vi "Test Bench v19 - prep.vi"(6 "Signal Output\nControl":enum32{"White Noise", "Harmonic"}(tab), 8 "Enable Display":bool=TRUE, 9 "Accel. 2":bool, 10 "Output":bool=TRUE) -> (2 "Accel. 1 Raw":dbl[](graph), 3 "Output Signal":dynamicdata(graph))   [LabVIEW 2022 SP3]
uses:
  <vilib>/Utility/error.llb/DialogType.ctl
  <vilib>/DAQmx/create/channels.llb/DAQmx Create Channel (AI-Acceleration-Accelerometer).vi
  <vilib>/DAQmx/create/channels.llb/DAQmx Create Channel (AO-Voltage-Basic).vi
  <vilib>/DAQmx/configure/timing.llb/DAQmx Timing (Sample Clock).vi
  <vilib>/DAQmx/miscellaneous.llb/DAQmx Fill In Error Info.vi
  WhiteNoise.ctl
  <vilib>/DAQmx/write.llb/DAQmx Write (Analog 2D DBL NChan NSamp).vi
  <vilib>/DAQmx/read.llb/DAQmx Read (Analog 1D DBL 1Chan NSamp).vi
  <vilib>/measure/NI_MABase.lvlib
panel:
  out "Input Data":dbl[](array[numeric])
  out "Output Data":dbl[](array[numeric])
  in  "White Noise\nParameters":T2={"Seed"=0.0, "Standard Deviation"=0.2, "Reset"=FALSE, "Iterator"=1.0, "Seed"=-1, "Lower Cut-Off"=5.0, "Upper Cut-Off"=350.0} {"Upper Cut-Off" min=5.0 max=350.0 step=10.0; "Lower Cut-Off" min=5.0 max=350.0 step=10.0; "Standard Deviation" min=0.001 max=3.0 step=0.05 format="%0.2p"}
  in  "Hamonic\nParameters":T3={"Waveform Type"=0, "Frequency"=10.0, "Amplitude"=0.25} {"Frequency" min=5.0 max=350.0 step=10.0 format="%0.2p"; "Waveform Type" items=["Sine Wave", "Triangle Wave", "Square Wave", "Sawtooth Wave"]; "Amplitude" min=0.001 max=0.3 step=0.05 format="%0.2p"}
  # "Filter"
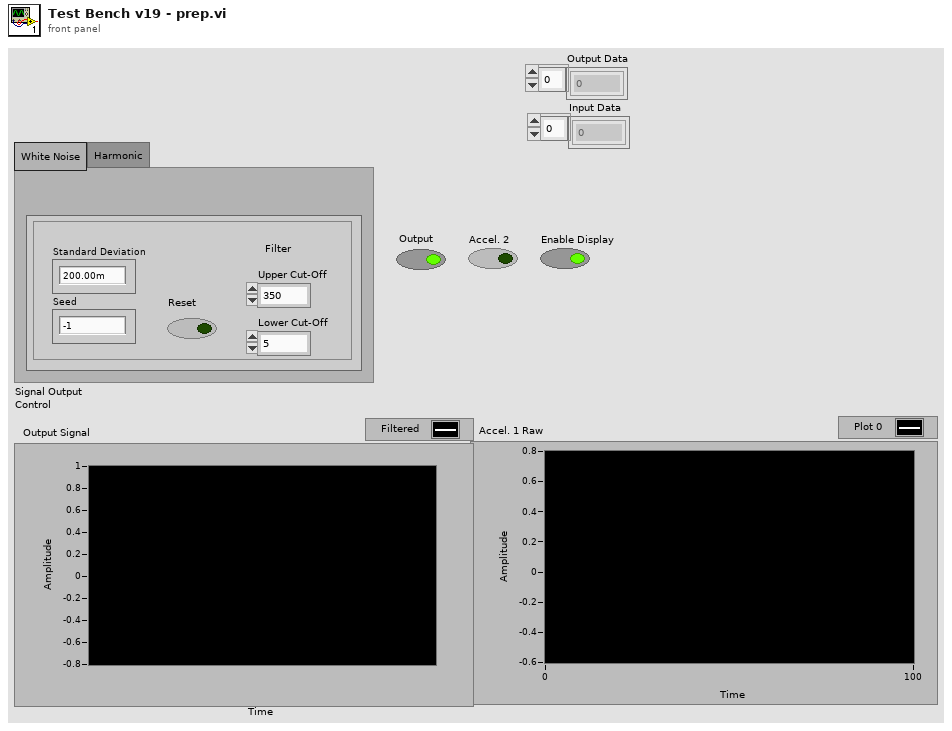
[diagram p1: front panel]
types:
  T1 = typedef "WhiteNoise.ctl" = dbl
  T2 = cluster{"Seed":T1, "Standard Deviation":dbl, "Reset":bool, "Iterator":dbl, "Seed":i8, "Lower Cut-Off":dbl, "Upper Cut-Off":dbl}
  T3 = cluster{"Waveform Type":u16, "Frequency":dbl, "Amplitude":dbl}
  T4 = typedef "DialogType.ctl" = u16
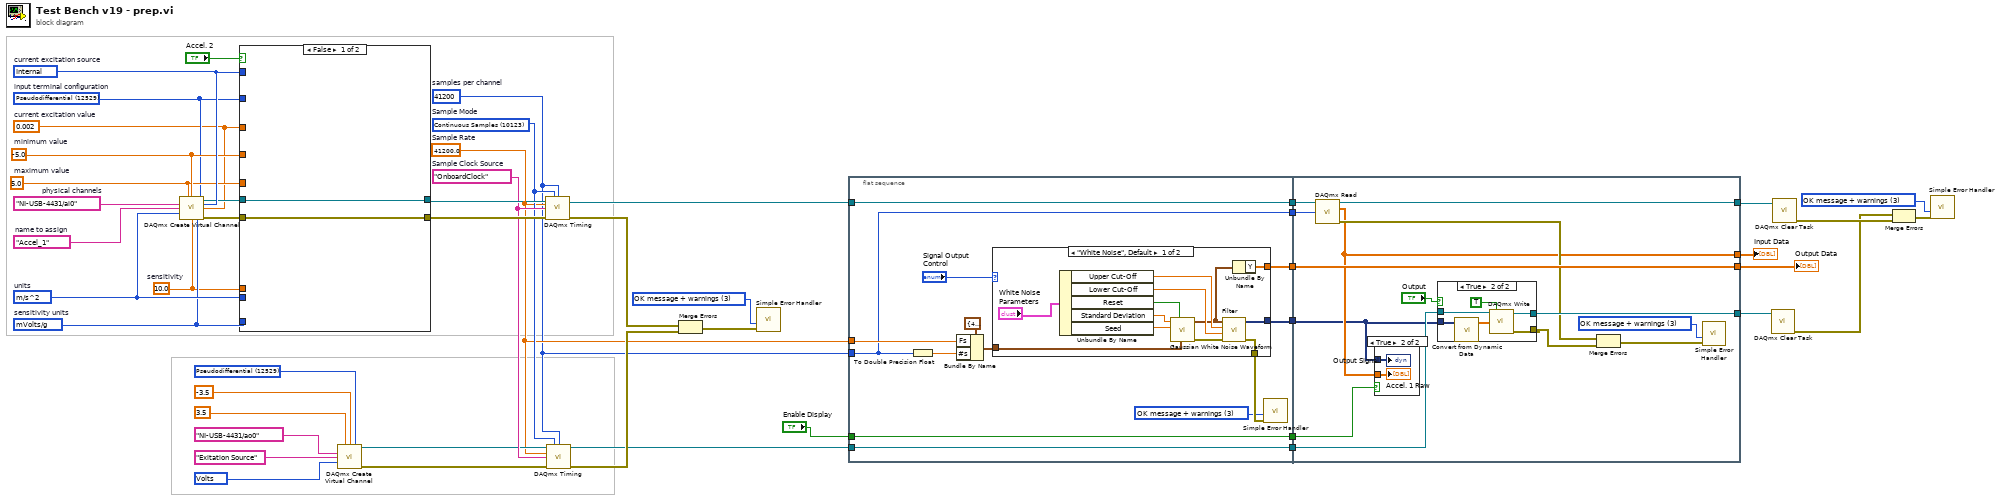
[diagram p0: block diagram]
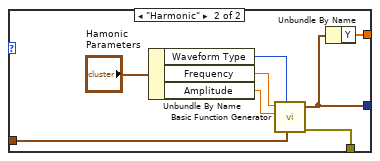
[diagram p2: hidden frame]
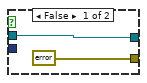
[diagram p4: hidden frame]
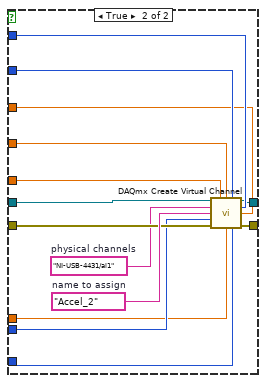
[diagram p5: hidden frame]
diagram:
  w9 = T4 3 items=["no dialog", "OK message", "continue or stop message", "OK message + warnings", "continue/stop + warnings"] ("type of dialog (OK msg:1)")
  w19 = T4 3 items=["no dialog", "OK message", "continue or stop message", "OK message + warnings", "continue/stop + warnings"] ("type of dialog (OK msg:1)")
  w15 = 41200  # samples per channel
  w35 = 12529 items=["Default"=-1, "RSE"=10083, "Differential"=10106, "Pseudodifferential"=12529] ("output terminal configuration")
  w33 = 10348 items=["Volts"=10348, "From Custom Scale"=10065] ("units")
  w39 = 12509 items=["mVolts/g"=12509, "Volts/g"=12510]  # sensitivity units
  w30 = 10.0  # sensitivity
  w38 = 0.002  # current excitation value
  w46 = 10200 items=["Internal"=10200, "External"=10167, "None"=10230]  # current excitation source
  w40 = tag "NI-USB-4431/ai0"  # physical channels
  w27 = tag "OnboardClock"  # Sample Clock Source
  w16 = 41200.0  # Sample Rate
  w26 = 10123 items=["Finite Samples"=10178, "Continuous Samples"=10123, "Hardware Timed Single Point"=12522]  # Sample Mode
  w42 = 12529 items=["default"=-1, "RSE"=10083, "NRSE"=10078, "Differential"=10106, "Pseudodifferential"=12529]  # input terminal configuration
  w45 = -5.0  # minimum value
  w44 = 5.0  # maximum value
  w48 = "Accel_1"  # name to assign
  w43 = 12470 items=["g"=10186, "m/s^2"=12470, "in/s^2"=12471, "From Custom Scale"=10065]  # units
  n1 = call-poly <vilib>:"DAQmx Create Virtual Channel.vi"("maximum value"=w44, "minimum value"=w45, "input terminal configuration"=w42, "physical channels"=w40, "current excitation source"=w46, "name to assign"=w48, "current excitation value"=w38, "units"=w43, "sensitivity"=w30, "sensitivity units"=w39) -> ("task out"=w41:refnum<k21>, "error out"=w47:errorcluster)  [unwired: 4 in]
  n2 = case shown="False" "Accel. 2" {
    tunnel: w47 -> [w50 w63]
    tunnel: w46 -> [_ w62]
    tunnel: w45 -> [_ w61]
    tunnel: w44 -> [_ w60]
    tunnel: w43 -> [_ w59]
    tunnel: w42 -> [_ w58]
    tunnel: w41 -> [w49 w57]
    tunnel: w39 -> [_ w55]
    tunnel: w38 -> [_ w54]
    tunnel: w30 -> [_ w53]
    tunnel: [w50 w52] -> w29
    tunnel: [w49 w51] -> w28
    frame False {
    }
    frame True {
      w56 = tag "NI-USB-4431/ai1"  # physical channels
      w64 = "Accel_2"  # name to assign
      n3 = call-poly <vilib>:"DAQmx Create Virtual Channel.vi"("task in"=w57, "maximum value"=w60, "minimum value"=w61, "input terminal configuration"=w58, "physical channels"=w56, "current excitation source"=w62, "name to assign"=w64, "current excitation value"=w54, "units"=w59, "error in"=w63, "sensitivity"=w53, "sensitivity units"=w55) -> ("task out"=w51:refnum<k21>, "error out"=w52:errorcluster)  [unwired: 2 in]
    }
  }
  n4 = call-poly <vilib>:"DAQmx Create Virtual Channel.vi"("maximum value"=3.5, "minimum value"=-3.5, "output terminal configuration"=w35, "physical channels"=tag "NI-USB-4431/ao0", "name to assign"="Exitation Source", "units"=w33) -> ("task out"=w24:refnum<k21>, "error out"=w25:errorcluster)  [unwired: 8 in]
  n5 = call-poly <vilib>:"DAQmx Timing.vi"("task/channels in"=w28, "sample mode"=w26, "samples per channel"=w15, "rate"=w16, "source"=w27, "error in"=w29) -> ("task out"=w18:refnum<k21>, "error out"=w32:errorcluster)  [unwired: 8 in]
  n6 = call-poly <vilib>:"DAQmx Timing.vi"("task/channels in"=w24, "sample mode"=w26, "samples per channel"=w15, "rate"=w16, "source"=w27, "error in"=w25) -> ("task out"=w22:refnum<k21>, "error out"=w23:errorcluster)  [unwired: 8 in]
  n7 = Merge Errors(w32, w23) -> (w17:errorcluster)
  n8 = call <vilib>:"Simple Error Handler.vi"("type of dialog (OK msg:1)"=w19, "error in (no error)"=w17) -> ()  [unwired: 3 in, 5 out]
  n9 = flat-sequence {
    tunnel: [w74] -> w14
    tunnel: [w70] -> w13
    tunnel: [w73] -> w12
    tunnel: [w71] -> w11
    tunnel: [w72] -> w10
    tunnel: w22 -> [w73]
    tunnel: w18 -> [w74]
    tunnel: "Enable Display" -> [w71]
    tunnel: w15 -> [w65]
    tunnel: w16 -> [w67]
    tunnel: [w65] -> w3
    tunnel: w14 -> [w104]
    tunnel: w13 -> [w111]
    tunnel: w12 -> [w109]
    tunnel: w11 -> [w105]
    tunnel: w10 -> [w98]
    tunnel: [w102] -> w7
    tunnel: [w111] -> w6
    tunnel: [w108] -> w4
    tunnel: [w106] -> w5
    tunnel: w3 -> [w103]
    frame #0 {
      w68 = T4 3 items=["no dialog", "OK message", "continue or stop message", "OK message + warnings", "continue/stop + warnings"] ("type of dialog (OK msg:1)")
      n10 = To Double Precision Float(number=w65) -> (double precision float=w66:dbl)
      n11 = Bundle By Name(cluster=cluster{"Fs":dbl, "#s":dbl} {"Fs"=41200.0, "#s"=41200.0} ("sampling info"), "Fs"=w67, "#s"=w66) -> (w76:cluster{"Fs":dbl, "#s":dbl})
      n12 = case shown="\"White Noise\", Default" "Signal Output\nControl" {
        tunnel: w76 -> [w87 w96]
        tunnel: [w80 w92] -> w72
        tunnel: [w79 w91] -> w70
        tunnel: [w78 w90] -> w69
        frame "White Noise", Default {
          n13 = Unbundle By Name("White Noise\nParameters") -> ("Upper Cut-Off"=w83:dbl, "Lower Cut-Off"=w82:dbl, "Reset"=w84:bool, "Standard Deviation"=w85:dbl, "Seed"=w86:T1)
          n14 = call <vilib>:"Gaussian White Noise Waveform.vi"("sampling info"=w87, "reset signal"=w84, "seed"=w86, "standard deviation"=w85) -> ("error out"=w89:errorcluster, "signal out"=w81:waveform(dbl))  [unwired: 6 in]
          n15 = call "Filter"("error in (no error)"=w89, "Lower Cut-Off"=w82, "Upper Cut-Off"=w83, "Signal"=w81) -> ("error out"=w78:errorcluster, "Filtered Signal"=w80:dynamicdata)  [unwired: 6 in]
          n16 = Unbundle By Name(w81) -> ("Y"=w79:dbl[])
        }
        frame "Harmonic" {
          n17 = Unbundle By Name("Hamonic\nParameters") -> ("Waveform Type"=w95:u16, "Frequency"=w94:dbl, "Amplitude"=w93:dbl)
          n18 = call <vilib>:"Basic Function Generator.vi"("sampling info"=w96, "signal type"=w95, "amplitude"=w93, "frequency"=w94) -> ("error out"=w90:errorcluster, "signal out"=w92:waveform(dbl))  [unwired: 5 in, 1 out]
          n19 = Unbundle By Name(w92) -> ("Y"=w91:dbl[])
        }
      }
      n20 = call <vilib>:"Simple Error Handler.vi"("type of dialog (OK msg:1)"=w68, "error in (no error)"=w69) -> ()  [unwired: 3 in, 5 out]
    }
    frame #1 {
      w101 = T4 3 items=["no dialog", "OK message", "continue or stop message", "OK message + warnings", "continue/stop + warnings"] ("type of dialog (OK msg:1)")
      n21 = call-poly <vilib>:"DAQmx Read.vi"("task/channels in"=w104, "number of samples per channel"=w103) -> ("task out"=w106:refnum<k21>, "data"=w102:dbl[], "error out"=w107:errorcluster)  [unwired: 11 in]
      n22 = case shown="True" w105 {
        tunnel: w102 -> [_ w113]
        tunnel: w98 -> [_ w112]
        frame False {
        }
        frame True {
          "Accel. 1 Raw" <- w113
          "Output Signal" <- w112
        }
      }
      n23 = case shown="True" "Output" {
        tunnel: w109 -> [w115 w121]
        tunnel: [errorcluster {"status"=FALSE, "code"=0, "source"=""} ("error out") w119] -> w100
        tunnel: [w115 w120] -> w108
        tunnel: w98 -> [_ w118]
        frame False {
        }
        frame True {
          n24 = call "Convert from Dynamic Data"("Dynamic Data Type"=w118) -> ("Array"=w117:dbl[][])  [unwired: 3 in]
          n25 = call-poly <vilib>:"DAQmx Write.vi"("task/channels in"=w121, "auto start"=TRUE, "data"=w117) -> ("task out"=w120:refnum<k21>, "error out"=w119:errorcluster)  [unwired: 10 in, 1 out]
        }
      }
      n26 = Merge Errors(w107, w100) -> (w99:errorcluster)
      n27 = call <vilib>:"Simple Error Handler.vi"("type of dialog (OK msg:1)"=w101, "error in (no error)"=w99) -> ()  [unwired: 3 in, 5 out]
    }
  }
  n28 = call <vilib>:"DAQmx Clear Task.vi"("task in"=w4) -> ("error out"=w2:errorcluster)  [unwired: 14 in]
  n29 = call <vilib>:"DAQmx Clear Task.vi"("task in"=w5) -> ("error out"=w8:errorcluster)  [unwired: 14 in]
  n30 = Merge Errors(w2, w8) -> (w1:errorcluster)
  n31 = call <vilib>:"Simple Error Handler.vi"("type of dialog (OK msg:1)"=w9, "error in (no error)"=w1) -> ()  [unwired: 3 in, 5 out]
  "Output Data" <- w6
  "Input Data" <- w7
